vi "Convert Data to DTC Frame.vi"(11 "Data":dbl[](array[numeric])) -> (3 "DTC Frame":u8[](array[numeric]) format="%.0b")   [LabVIEW 2013, in "J1939 Addon Engine.lvlib"]
uses:
  J1939 Addon Engine.lvlib
  Shared/Types/Convert DTCs Cluster.ctl
  Shared/J1939 Addon Shared.lvlib
panel:
  in  "Cluster 2":T1
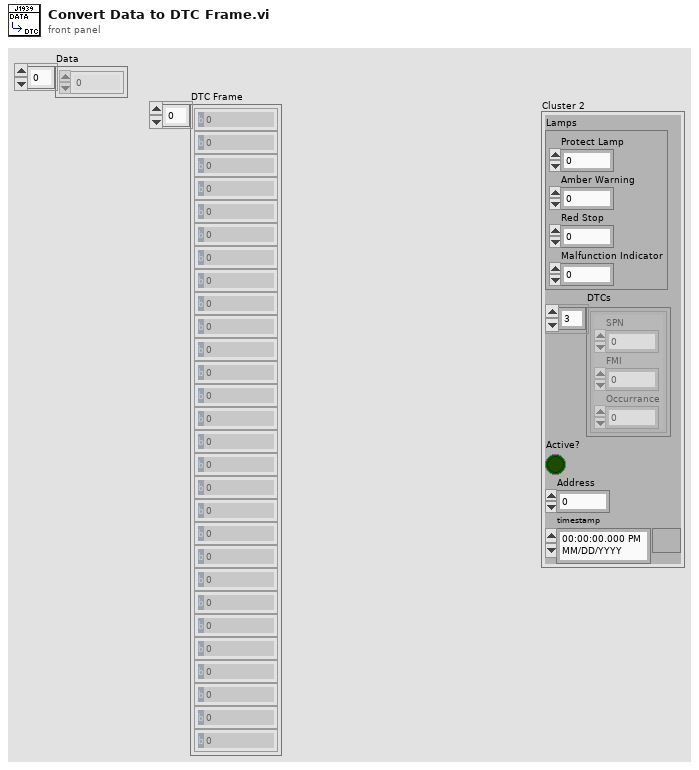
[diagram p1: front panel]
types:
  T1 = typedef "J1939 Addon Shared.lvlib/Convert DTCs Cluster.ctl" = cluster{"Lamps":cluster{"Protect Lamp":u8, "Amber Warning":u8, "Red Stop":u8, "Malfunction Indicator":u8}, "DTCs":cluster{"SPN":u32, "FMI":u8, "Occurrance":u8}[], "Active?":bool, "Address":u8, "timestamp":timestamp}
  T2 = cluster{"Protect Lamp":u8, "Amber Warning":u8, "Red Stop":u8, "Malfunction Indicator":u8}
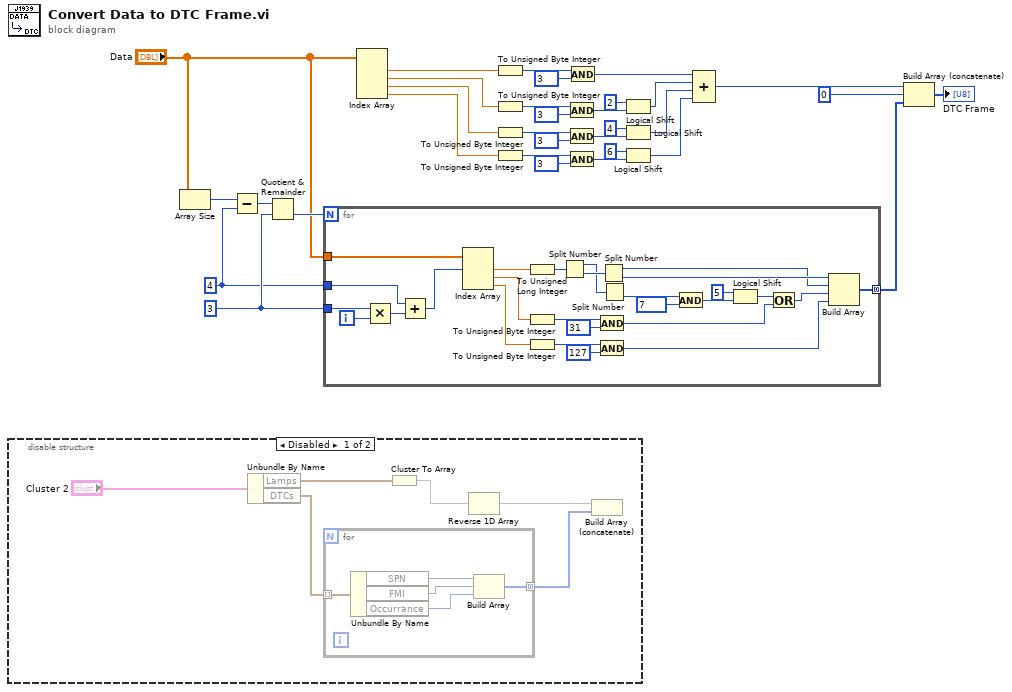
[diagram p0: block diagram]
diagram:
  w4 = 3 ("x")
  w3 = 4 ("x")
  n1 = disable-structure shown="Disabled" {
    frame Disabled {
      n2 = Unbundle By Name("Cluster 2") -> ("Lamps"=w37:T2, "DTCs"=w36:cluster{"SPN":u32, "FMI":u8, "Occurrance":u8}[])
      n3 = for {
        tunnel: w36 -> [w43] mode=indexing
        tunnel: [w39] -> w34 mode=concatenating
        n4 = Unbundle By Name(w43) -> ("SPN"=w42:u32, "FMI"=w41:u8, "Occurrance"=w40:u8)
        n5 = Build Array(w42, w41, w40) -> (w39:u32[])
      }
      n6 = Cluster To Array(cluster=w37) -> (array=w35:u8[])
      n7 = Reverse 1D Array(array=w35) -> (reversed array=w33:u8[])
      n8 = Build Array (concatenate)(w33, w34) -> ()  [unwired: 1 out]
    }
    frame Enabled {
    }
  }
  n9 = Array Size(array="Data") -> (size(s)=w7:i32)
  n10 = Subtract(x=w7, y=w3) -> (x-y=w8:i32)
  n11 = Quotient & Remainder(x=w8, y=w4) -> (floor(x/y)=w5:i32)  [unwired: 1 out]
  n12 = for {
    N: w5 -> [_]
    tunnel: "Data" -> [w57]
    tunnel: [w49] -> w6 mode=concatenating
    tunnel: w4 -> [w47]
    tunnel: w3 -> [w45]
    i -> [w48]
    n13 = Multiply(x=w47, y=w48) -> (x*y=w46:i32)
    n14 = Add(x=w45, y=w46) -> (x+y=w44:i32)
    n15 = Index Array(array=w57, index #1=w44) -> (element #1=w56:dbl, element #2=w55:dbl, element #3=w54:dbl)  [unwired: 2 in]
    n16 = To Unsigned Long Integer(number=w56) -> (unsigned 32bit integer=w70:u32)
    n17 = To Unsigned Byte Integer(number=w55) -> (unsigned 8bit integer=w62:u8)
    n18 = To Unsigned Byte Integer(number=w54) -> (unsigned 8bit integer=w64:u8)
    n19 = Split Number(x=w70) -> (hi(x)=w68:u16, lo(x)=w69:u16)
    n20 = And(x=w62, y=u8 31) -> (x .and. y?=w58:u8)
    n21 = And(x=w64, y=u8 127) -> (x .and. y?=w50:u8)
    n22 = Split Number(x=w69) -> (hi(x)=w52:u8, lo(x)=w53:u8)
    n23 = Split Number(x=w68) -> (lo(x)=w66:u8)  [unwired: 1 out]
    n24 = And(x=w66, y=u8 7) -> (x .and. y?=w61:u8)
    n25 = Logical Shift(y=i16 5, x=w61) -> (x << y=w59:u8)
    n26 = Or(x=w59, y=w58) -> (x .or. y?=w51:u8)
    n27 = Build Array(w53, w52, w51, w50) -> (w49:u8[])
  }
  n28 = Index Array(array="Data") -> (element #1=w32:dbl, element #2=w23:dbl, element #3=w22:dbl, element #4=w21:dbl)  [unwired: 4 in]
  n29 = To Unsigned Byte Integer(number=w32) -> (unsigned 8bit integer=w31:u8)
  n30 = To Unsigned Byte Integer(number=w23) -> (unsigned 8bit integer=w28:u8)
  n31 = To Unsigned Byte Integer(number=w22) -> (unsigned 8bit integer=w27:u8)
  n32 = To Unsigned Byte Integer(number=w21) -> (unsigned 8bit integer=w24:u8)
  n33 = And(x=w28, y=u8 3) -> (x .and. y?=w19:u8)
  n34 = And(x=w27, y=u8 3) -> (x .and. y?=w18:u8)
  n35 = And(x=w24, y=u8 3) -> (x .and. y?=w20:u8)
  n36 = And(x=w31, y=u8 3) -> (x .and. y?=w14:u8)
  n37 = Logical Shift(y=i16 2, x=w19) -> (x << y=w13:u8)
  n38 = Logical Shift(y=i16 4, x=w18) -> (x << y=w12:u8)
  n39 = Logical Shift(y=i16 6, x=w20) -> (x << y=w11:u8)
  n40 = Compound Arithmetic op=ADD(w14, w13, w12, w11) -> (w10:u8)
  n41 = Build Array (concatenate)(w10, u8 0 ("element"), w6) -> (→"DTC Frame":u8[])
